vi "setDoubleField.vi"(8 "error in (no error)":errorcluster, 11 "PulseData in":refnum<class "PulseData.lvclass">) -> (0 "error out":errorcluster, 3 "PulseData out":refnum<class "PulseData.lvclass">)   [LabVIEW 2013, in "Controls Log Monitor.lvlib" / "PulseData.lvclass"]
uses:
  PulseData.lvclass
  PulseData.lvclass/PulseData.ctl
panel:
  in  "Value String":string
  in  "Field Name":string
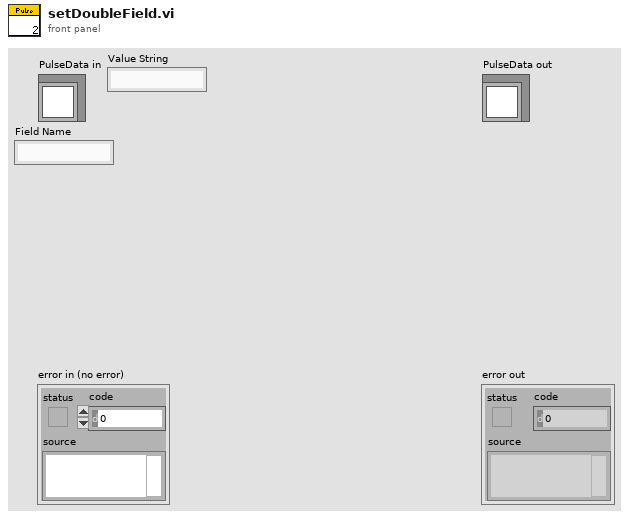
[diagram p1: front panel]
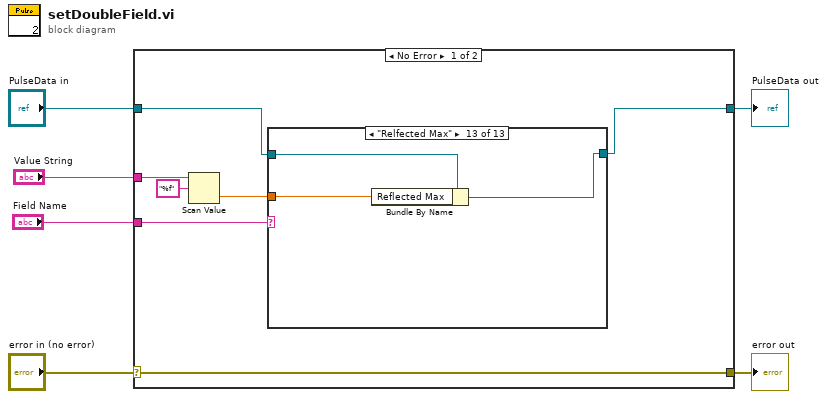
[diagram p0: block diagram]
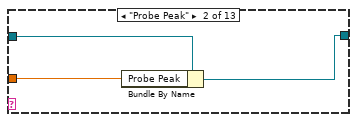
[diagram p3: hidden frame]
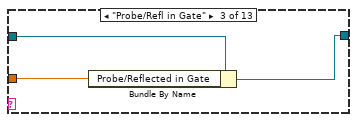
[diagram p4: hidden frame]
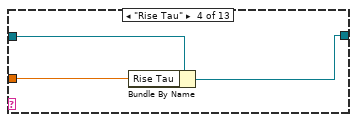
[diagram p5: hidden frame]
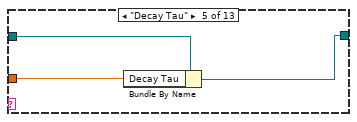
[diagram p6: hidden frame]
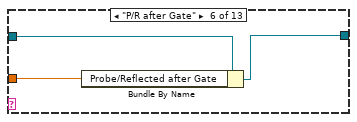
[diagram p7: hidden frame]
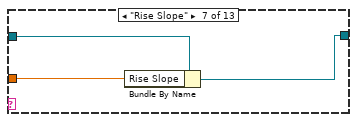
[diagram p8: hidden frame]
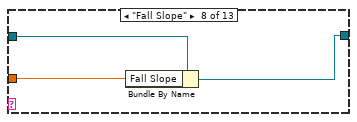
[diagram p9: hidden frame]
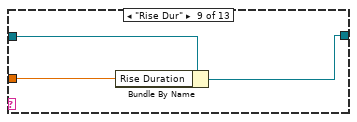
[diagram p10: hidden frame]
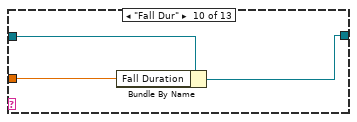
[diagram p11: hidden frame]
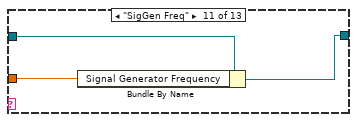
[diagram p12: hidden frame]
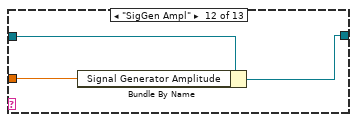
[diagram p13: hidden frame]
diagram:
  n1 = case shown="No Error" "error in (no error)" {
    selector: "error in (no error)" -> [w13 w52]
    tunnel: [w13 w52] -> w5
    tunnel: [w8 w51] -> w3
    tunnel: "PulseData in" -> [w12 w51]
    tunnel: "Field Name" -> [w11 _]
    tunnel: "Value String" -> [w7 _]
    frame No Error {
      n2 = Scan Value(string=w7, format string="%f") -> (value=w9:dbl)  [unwired: 1 in, 1 out]
      n3 = case shown="\"Relfected Max\"" w11 {
        tunnel: w12 -> [w14 w17 w20 w23 w26 w29 w32 w35 w38 w41 w44 w47 w50]
        tunnel: w9 -> [_ w16 w19 w22 w25 w28 w31 w34 w37 w40 w43 w46 w49]
        tunnel: [w14 w15 w18 w21 w24 w27 w30 w33 w36 w39 w42 w45 w48] -> w8
        frame Default {
        }
        frame "Probe Peak" {
          n4 = Bundle By Name(cluster=w17, "Probe Peak"=w16) -> (w15:refnum<class "PulseData.lvclass">)
        }
        frame "Probe/Refl in Gate" {
          n5 = Bundle By Name(cluster=w20, "Probe/Reflected in Gate"=w19) -> (w18:refnum<class "PulseData.lvclass">)
        }
        frame "Rise Tau" {
          n6 = Bundle By Name(cluster=w23, "Rise Tau"=w22) -> (w21:refnum<class "PulseData.lvclass">)
        }
        frame "Decay Tau" {
          n7 = Bundle By Name(cluster=w26, "Decay Tau"=w25) -> (w24:refnum<class "PulseData.lvclass">)
        }
        frame "P/R after Gate" {
          n8 = Bundle By Name(cluster=w29, "Probe/Reflected after Gate"=w28) -> (w27:refnum<class "PulseData.lvclass">)
        }
        frame "Rise Slope" {
          n9 = Bundle By Name(cluster=w32, "Rise Slope"=w31) -> (w30:refnum<class "PulseData.lvclass">)
        }
        frame "Fall Slope" {
          n10 = Bundle By Name(cluster=w35, "Fall Slope"=w34) -> (w33:refnum<class "PulseData.lvclass">)
        }
        frame "Rise Dur" {
          n11 = Bundle By Name(cluster=w38, "Rise Duration"=w37) -> (w36:refnum<class "PulseData.lvclass">)
        }
        frame "Fall Dur" {
          n12 = Bundle By Name(cluster=w41, "Fall Duration"=w40) -> (w39:refnum<class "PulseData.lvclass">)
        }
        frame "SigGen Freq" {
          n13 = Bundle By Name(cluster=w44, "Signal Generator Frequency"=w43) -> (w42:refnum<class "PulseData.lvclass">)
        }
        frame "SigGen Ampl" {
          n14 = Bundle By Name(cluster=w47, "Signal Generator Amplitude"=w46) -> (w45:refnum<class "PulseData.lvclass">)
        }
        frame "Relfected Max" {
          n15 = Bundle By Name(cluster=w50, "Reflected Max"=w49) -> (w48:refnum<class "PulseData.lvclass">)
        }
      }
    }
    frame Error {
    }
  }
  "error out" <- w5
  "PulseData out" <- w3
